vi "Read.vi"(8 "error in (no error)":errorcluster caption="entrée d'erreur (pas d'erreur)", 11 "Class DIO (Default) en entrée":refnum<class "Class DIO NI.lvclass">) -> (0 "error out":errorcluster caption="sortie d'erreur", 3 "Class DIO (Default) en sortie":refnum<class "Class DIO NI.lvclass">)   [LabVIEW 2020, in "Library Instrument & Equipement.lvlib" / "Library DIO.lvlib" / "Class DIO NI.lvclass"]
uses:
  Class DIO NI.lvclass
  C:/Users/ngarcin/OneDrive - Altyor/Standard TB/Class/DIO/Class DIO (Default)/Class DIO (Default).lvclass
  Commun VI/TypeDef/Liste Error.ctl
  <vilib>/DAQmx/read.llb/DAQmx Read (Digital Bool 1Line 1Point).vi
  <vilib>/DAQmx/miscellaneous.llb/DAQmx Fill In Error Info.vi
  Class DIO NI.lvclass/Class DIO NI.ctl
  Commun VI/Library Commun.lvlib
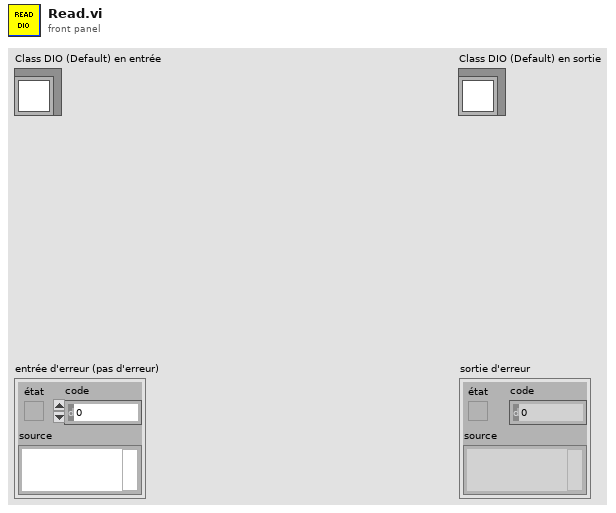
[diagram p1: front panel]
types:
  T1 = typedef "Library Commun.lvlib/Liste Error.ctl" = enum16{"Firebase Driver - Get Document", "Firebase Driver - Get Document With Where", "Firebase Driver - Delete Document", "Firebase Driver - Set Document", "Firebase Driver - Update Document", "Firebase Altyor - Search Document Bench", "Firebase Altyor - Class Not in Firebase", "Spectrum_Analyser - Timeout", "Relay Board - Qty Relay", "DIO - Pb Funtion", "Power_Supply - Peripherical not find", "Mutimeter - Peripherical not find", "Instrument - Function Not Used", "Instrument - Instrument name not specified", "Instrument - Allready Initialised", "Instrument - TimeOut", "Instrument - the instrument must be Initialise before", "Instrument - Frame Not received", "Instrument - Frame Nok", "Test - Initialise the File_for_Save", "Test - Timeout", "Test - Cmd Error", "FGV - Variable ", "BDD FireBase - Define Class", "SN - Class Not Define"}
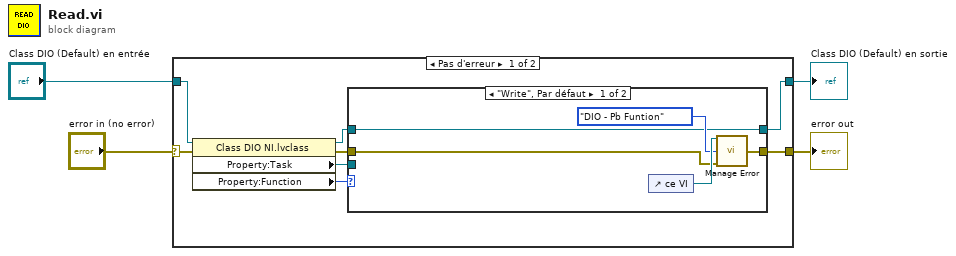
[diagram p0: block diagram]
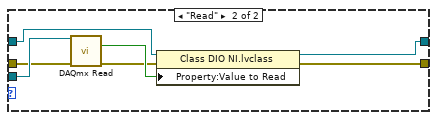
[diagram p2: hidden frame]
diagram:
  n1 = case shown="Pas d'erreur" "error in (no error)" {
    selector: "error in (no error)" -> [w9 w26]
    tunnel: [w8 w26] -> w3
    tunnel: [w6 w25] -> w1
    tunnel: "Class DIO (Default) en entrée" -> [w12 w25]
    frame No Error {
      n2 = property class="Class DIO NI.lvclass"(reference=w12, error in=w9) -> (reference out=w7:refnum<class "Class DIO NI.lvclass">, error out=w10:errorcluster, "Property:Task"=w11:refnum<k21>, "Property:Function"=w5:enum16{"Write", "Read"})
      n3 = case shown="\"Write\", Par défaut" w5 {
        tunnel: w11 -> [_ w24]
        tunnel: w10 -> [w13 w23]
        tunnel: [w14 w20] -> w8
        tunnel: w7 -> [w15 w19]
        tunnel: [w15 w18] -> w6
        frame "Write", Default {
          n4 = control-ref of="ce VI"() -> (w17:refnum<vi>)
          n5 = call "Manage Error.vi"("VI in Error"=w17, "Code Erreur"=Liste_Error."DIO - Pb Funtion", "error in (no error)"=w13) -> ("error out"=w14:errorcluster)  [unwired: 12 in]
        }
        frame "Read" {
          n6 = call-poly <vilib>:"DAQmx Read.vi"("task/channels in"=w24, "error in"=w23) -> ("data"=w22:bool, "error out"=w21:errorcluster)  [unwired: 11 in, 1 out]
          n7 = property class="Class DIO NI.lvclass"(reference=w19, error in=w21, "Property:Value to Read"=w22) -> (reference out=w18:refnum<class "Class DIO NI.lvclass">, error out=w20:errorcluster)
        }
      }
    }
    frame Error {
    }
  }
  "error out" <- w3
  "Class DIO (Default) en sortie" <- w1
